vi "Convert C to F.vi"(1 "Temp in C":dbl) -> (0 "Temp in F":dbl)   [LabVIEW 2010]
uses:
  <vilib>/express/express arith-compare/Formula/XNode/ExpressFormulaBlockNode.xnode
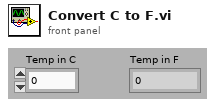
[diagram p1: front panel]
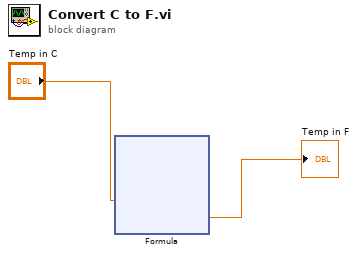
[diagram p0: block diagram]
diagram:
  n1 = xnode "Formula"("X1"="Temp in C") -> ("Result"=→"Temp in F":dbl)  [unwired: 1 in, 1 out]
